vi "image size-related calculation.vi"(11 "Refnum in":T1) -> (0 "height less than 1cm(80pixels)":bool, 2 "width":i32, 3 "no. of scanning lines":i32)   [LabVIEW 2011]
uses:
  <vilib>/vision/Image Controls.llb/IMAQ Image.ctl
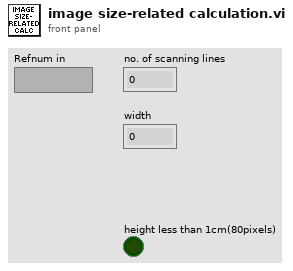
[diagram p1: front panel]
types:
  T1 = typedef "IMAQ Image.ctl" = refnum<image>
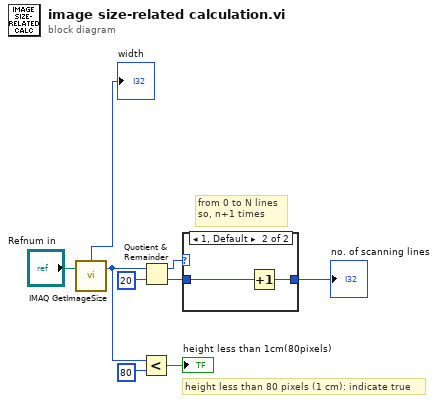
[diagram p0: block diagram]
diagram:
  # "height less than 80 pixels (1 cm): indicate true"
  # "from 0 to N lines\nso, n+1 times"
  n1 = call "IMAQ GetImageSize"("Image"="Refnum in") -> ("Y Resolution"=w8:i32, "X Resolution"=→"width":i32)  [unwired: 3 in, 1 out]
  n2 = Less?(x=w8, y=80) -> (x < y?=→"height less than 1cm(80pixels)":bool)
  n3 = Quotient & Remainder(x=w8, y=20) -> (x-y*floor(x/y)=w9:i32, floor(x/y)=w3:i32)
  n4 = case shown="1, Default" w9 {
    tunnel: w3 -> [w10 w12]
    tunnel: [w10 w11] -> w4
    frame 0 {
    }
    frame 1, Default {
      n5 = Increment(x=w12) -> (x+1=w11:i32)
    }
  }
  "no. of scanning lines" <- w4
